vi "Teleop.vi"(10 "Match Info":T1={"Autonomous Elapsed Seconds"=0.0, "TeleOp Elapsed Seconds"=0.0, "Disabled Elapsed Seconds"=0.0, "Visited Autonomous"=FALSE, "Visited TeleOp"=FALSE, "Visited Disabled"=FALSE, "Autonomous Settings"={"Autonomous Style"=enum."Independent", "VI Refnum"=refnum}}, 11 "Call Context":T2) -> ()   [LabVIEW 2017]
doc: "This VI is called for each TeleOp packet received from the DS where the robot is not disabled. It is often used to read from the joysticks and update I/O or to update setpoints for timed control loops. It should complete and return within 20 milliseconds or it may miss DS packets."
uses:
  <vilib>/Rock Robotics/Network Tables/NT Write Numeric Array.vi
  <vilib>/Rock Robotics/Network Tables/NT Write Boolean Array.vi
  <vilib>/Rock Robotics/Network Tables/NT Read Boolean.vi
  <vilib>/Rock Robotics/Network Tables/NT Read Number.vi
  <vilib>/Rock Robotics/WPI/Solenoid/WPI_SolenoidValue.ctl
  <vilib>/Rock Robotics/WPI/Solenoid/WPI_SolenoidSetEnum.vi
  <vilib>/Rock Robotics/Network Tables/NT Write Boolean.vi
  <vilib>/Rock Robotics/WPI/DriverStation/WPI_DriverStationMatch Info.ctl
  <vilib>/Rock Robotics/WPI/DriverStation/WPI_DriverStationDerivedRobotMode.ctl
panel:
  out "Sample Slider 0":dbl(slide) scale=0.0..5.0
  out "Sample Boolean 1":bool
  out "Sample Boolean 0":bool
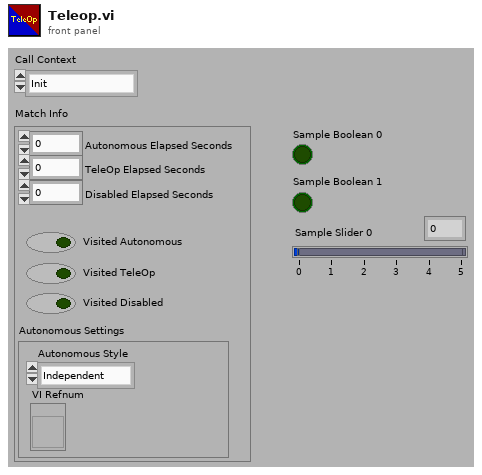
[diagram p1: front panel]
types:
  T1 = typedef "WPI_DriverStationMatch Info.ctl" = cluster{"Autonomous Elapsed Seconds":dbl, "TeleOp Elapsed Seconds":dbl, "Disabled Elapsed Seconds":dbl, "Visited Autonomous":bool, "Visited TeleOp":bool, "Visited Disabled":bool, "Autonomous Settings":cluster{"Autonomous Style":enum16{"Iterative", "Independent"}, "VI Refnum":refnum<vi>}}
  T2 = typedef "WPI_DriverStationDerivedRobotMode.ctl" = enum16{"Init", "Execute", "Stop"}
  T3 = enum16{"Piston", "na1", "na2", "na3", "na4", "na5", "na6", "Tapis_3_avancer", "Tapis_3_reculer", "Tapis_2_avancer", "Tapis_2_reculer", "Tapis_1_avancer", "Tapis_1_reculer"}
  T4 = typedef "WPI_SolenoidValue.ctl" = enum16{"Off", "On", "Forward", "Reverse"}
  T5 = typedef "WPI_RobotDriveDevRef.ctl" = cluster{"DevStatus":errorcluster, "Motors[]":T6[], "Square Inputs":bool, "Max Output":dbl}
  T6 = typedef "WPI_MotorControlDeviceRef.ctl" = cluster{"DeviceStatus":errorcluster, "Type":T7, "PWM":cluster{"PWM Channel":T8, "DeadBand":T9}, "CAN":cluster{"Device Number":u8, "SetOutput VI Ref":variant, "GetOutput VI Ref":variant, "Enable VI Ref":variant, "Disable VI Ref":variant, "Data":variant}, "Invert":bool, "DIO PWM":cluster{"PWM \"Enable\" Channel":T8, "DIOChannel":T10, "PWM Rate":dbl}}
  T7 = typedef "WPI_MotorControlType.ctl" = enum16{"PWM", "CAN", "DIO PWM"}
  T8 = typedef "FPGA_DIOPWMChannel.ctl" = enum8{"PWM 0", "PWM 1", "PWM 2", "PWM 3", "PWM 4", "PWM 5", "PWM 6", "PWM 7", "PWM 8", "PWM 9", "PWM MXP 0", "PWM MXP 1", "PWM MXP 2", "PWM MXP 3", "PWM MXP 4", "PWM MXP 5", "PWM MXP 6", "PWM MXP 7", "PWM MXP 8", "PWM MXP 9", "Invalid"}
  T9 = typedef "WPI_PWMDeadband.ctl" = cluster{"Name":string, "maxPositivePwm":i32, "minPositivePwm":i32, "centerPwm":i32, "maxNegativePwm":i32, "minNegativePwm":i32, "angularRange":u16}
  T10 = typedef "FPGA_DIOChannel.ctl" = enum8{"DIO 0", "DIO 1", "DIO 2", "DIO 3", "DIO 4", "DIO 5", "DIO 6", "DIO 7", "DIO 8", "DIO 9", "DIO MXP 0", "DIO MXP 1", "DIO MXP 2", "DIO MXP 3", "DIO MXP 4", "DIO MXP 5", "DIO MXP 6", "DIO MXP 7", "DIO MXP 8", "DIO MXP 9", "DIO MXP 10", "DIO MXP 11", "DIO MXP 12", "DIO MXP 13", "DIO MXP 14", "DIO MXP 15", "SPI Port CS1", "SPI Port CS2", "SPI Port CS3", "SPI Port MISO", "SPI Port MOSI", "Invalid"}
  T11 = typedef "WPI_JoystickDevRef.ctl" = cluster{"Device":T12}
  T12 = typedef "WPI_JoystickDeviceEnum.ctl" = enum16{"USB 0", "USB 1", "USB 2", "USB 3", "USB 4", "USB 5"}
  T13 = typedef "WPI_SolenoidDevRef.ctl" = cluster{"DevStatus":errorcluster, "Pneumatics Control Module":u8, "Forward Solenoid Channel":T14, "Reverse Solenoid Channel":T14}
  T14 = typedef "WPI_SolenoidChannel.ctl" = enum8{"Solenoid 0", "Solenoid 1", "Solenoid 2", "Solenoid 3", "Solenoid 4", "Solenoid 5", "Solenoid 6", "Solenoid 7", "Invalid"}
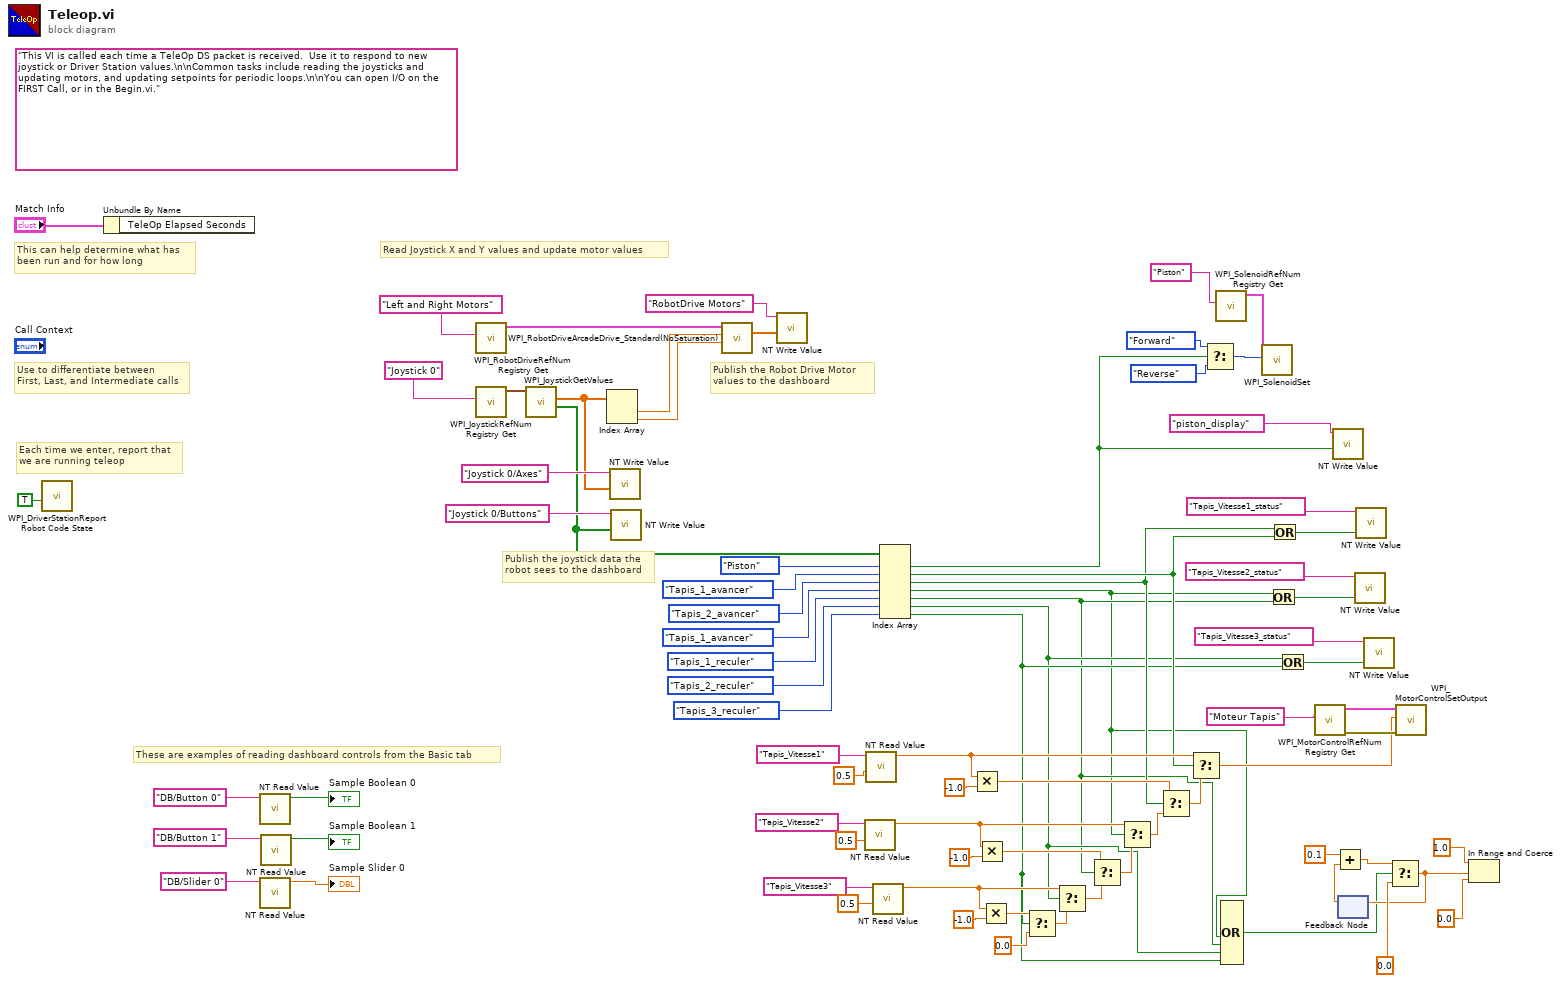
[diagram p0: block diagram]
diagram:
  (unwired) "This VI is called each time a TeleOp DS packet is received.  Use it to respond to new joystick or Driver Station values.\n\nCommon tasks include reading the joysticks and updating motors, and updating setpoints for periodic loops.\n\nYou can open I/O on the FIRST Call, or in the Begin.vi."
  # "These are examples of reading dashboard controls from the Basic tab"
  # "Publish the Robot Drive Motor\nvalues to the dashboard"
  # "Publish the joystick data the\nrobot sees to the dashboard"
  # "Each time we enter, report that\nwe are running teleop"
  # "Use to differentiate between\nFirst, Last, and Intermediate calls"
  # "This can help determine what has\nbeen run and for how long"
  # "Read Joystick X and Y values and update motor values"
  n1 = call <vilib>:"WPI_DriverStationReport Robot Code State.vi"("TeleOp"=TRUE ("Autonomous")) -> ()  [unwired: 10 in, 1 out]
  n2 = Unbundle By Name("Match Info") -> ()  [unwired: 1 out]
  n3 = call-poly <vilib>:"NT Read Value.vi"("Name"="DB/Button 0" ("refnum name")) -> ("Boolean"=→"Sample Boolean 0":bool)  [unwired: 9 in, 1 out]
  n4 = call-poly <vilib>:"NT Read Value.vi"("Name"="DB/Slider 0" ("refnum name")) -> ("Numeric"=→"Sample Slider 0":dbl)  [unwired: 9 in, 1 out]
  n5 = call-poly <vilib>:"NT Read Value.vi"("Name"="DB/Button 1" ("refnum name")) -> ("Boolean"=→"Sample Boolean 1":bool)  [unwired: 9 in, 1 out]
  n6 = call <vilib>:"WPI_RobotDriveRefNum Registry Get.vi"("refnum name"="Left and Right Motors") -> ("RobotDriveDevRef"=w77:T5)  [unwired: 1 in, 9 out]
  n7 = call <vilib>:"WPI_JoystickRefNum Registry Get.vi"("refnum name"="Joystick 0") -> ("JoystickDevRef"=w74:T11)  [unwired: 1 in, 9 out]
  n8 = call <vilib>:"WPI_JoystickGetValues.vi"("JoystickDevRef"=w74) -> ("Buttons"=w52:bool[], "Axes"=w69:dbl[])  [unwired: 6 in, 3 out]
  n9 = Index Array(array=w69) -> (element #1=w76:dbl, element #2=w72:dbl)  [unwired: 2 in]
  n10 = call-poly <vilib>:"NT Write Value.vi"("Numeric Array"=w69, "Name"="Joystick 0/Axes") -> ()  [unwired: 9 in, 1 out]
  n11 = call-poly <vilib>:"NT Write Value.vi"("Boolean Array"=w52, "Name"="Joystick 0/Buttons") -> ()  [unwired: 9 in, 1 out]
  n12 = call <vilib>:"WPI_RobotDriveArcadeDrive_Standard(NoSaturation).vi"("Y axis value"=w72, "X axis value"=w76, "RobotDriveDevRef"=w77) -> ("Motor Values"=w62:dbl[])  [unwired: 1 in, 7 out]
  n13 = call-poly <vilib>:"NT Write Value.vi"("Numeric Array"=w62, "Name"="RobotDrive Motors") -> ()  [unwired: 9 in, 1 out]
  n14 = call-poly <vilib>:"NT Read Value.vi"("Default Value"=0.5, "Name"="Tapis_Vitesse2") -> ("Numeric"=w29:dbl)  [unwired: 8 in, 1 out]
  n15 = call-poly <vilib>:"NT Read Value.vi"("Default Value"=0.5, "Name"="Tapis_Vitesse1") -> ("Numeric"=w24:dbl)  [unwired: 8 in, 1 out]
  n16 = call-poly <vilib>:"NT Read Value.vi"("Default Value"=0.5, "Name"="Tapis_Vitesse3") -> ("Numeric"=w33:dbl)  [unwired: 8 in, 1 out]
  n17 = Index Array(array=w52, index #1=T3."Piston", index #2=T3."Tapis_1_avancer", index #3=T3."Tapis_2_avancer", index #4=T3."Tapis_1_avancer", index #5=T3."Tapis_1_reculer", index #6=T3."Tapis_2_reculer", index #7=T3."Tapis_3_reculer") -> (element #1=w13:bool, element #2=w20:bool, element #3=w19:bool, element #4=w2:bool, element #5=w3:bool, element #6=w4:bool, element #7=w5:bool)
  n18 = Multiply(x=w24, y=-1.0) -> (x*y=w26:dbl)
  n19 = Multiply(x=w29, y=-1.0) -> (x*y=w30:dbl)
  n20 = Multiply(x=w33, y=-1.0) -> (x*y=w35:dbl)
  n21 = Select(t=w35, s=w5, f=0.0) -> (s? t:f=w34:dbl)
  n22 = Select(t=w33, s=w4, f=w34) -> (s? t:f=w31:dbl)
  n23 = Select(t=w30, s=w3, f=w31) -> (s? t:f=w32:dbl)
  n24 = Select(t=w29, s=w2, f=w32) -> (s? t:f=w25:dbl)
  n25 = Select(t=w26, s=w19, f=w25) -> (s? t:f=w27:dbl)
  n26 = Select(t=w24, s=w20, f=w27) -> (s? t:f=w23:dbl)
  n27 = Select(t=WPI_SolenoidValue."Forward" ("Value"), s=w13, f=WPI_SolenoidValue."Reverse" ("Value")) -> (s? t:f=w59:T4)
  n28 = call <vilib>:"WPI_SolenoidRefNum Registry Get.vi"("refnum name"="Piston") -> ("SolenoidDevRef"=w56:T13)  [unwired: 9 in, 1 out]
  n29 = Compound Arithmetic op=OR(w2, w3, w4, w5) -> (w1:bool)  [unwired: 4 in]
  n30 = call-poly <vilib>:"WPI_SolenoidSet.vi"("Value"=w59, "SolenoidDevRef"=w56) -> ()  [unwired: 1 in, 9 out]
  n31 = Or(x=w2, y=w3) -> (x .or. y?=w17:bool)
  n32 = Or(x=w19, y=w20) -> (x .or. y?=w21:bool)
  n33 = Or(x=w4, y=w5) -> (x .or. y?=w15:bool)
  n34 = call <vilib>:"WPI_MotorControlRefNum Registry Get.vi"("refnum name"="Moteur Tapis") -> ("error out"=w53:errorcluster, "MotorControlDevRef"=w54:T6)  [unwired: 9 in]
  n35 = call-poly <vilib>:"NT Write Value.vi"("Boolean"=w13, "Name"="piston_display") -> ()  [unwired: 9 in, 1 out]
  n36 = feedback #1() -> (w12:dbl)  [unwired: 1 in]
  n37 = Add(x=0.1, y=w12) -> (x+y=w10:dbl)
  n38 = call-poly <vilib>:"NT Write Value.vi"("Boolean"=w17, "Name"="Tapis_Vitesse2_status") -> ()  [unwired: 9 in, 1 out]
  n39 = call-poly <vilib>:"NT Write Value.vi"("Boolean"=w21, "Name"="Tapis_Vitesse1_status") -> ()  [unwired: 9 in, 1 out]
  n40 = call-poly <vilib>:"NT Write Value.vi"("Boolean"=w15, "Name"="Tapis_Vitesse3_status") -> ()  [unwired: 9 in, 1 out]
  n41 = Select(t=w10, s=w1, f=0.0) -> (s? t:f=w6:dbl)
  n42 = feedback-in #1(w6) -> ()
  n43 = call <vilib>:"WPI_MotorControlSetOutput.vi"("error in (no error)"=w53, "Output"=w23, "MotorControlDevRef"=w54) -> ()  [unwired: 6 in, 3 out]
  n44 = In Range and Coerce(upper limit=1.0, x=w6, lower limit=0.0) -> ()  [unwired: 2 out]
